vi "Get Target IP and Name.vi"(8 "error in (no error)":errorcluster, 11 "Item Ref in":T1 format="%.0x") -> (0 "error out":errorcluster, 1 "Name":string, 2 "IPAddress":string, 3 "Item Ref out":T1=18446744073709551615 format="%.0x")   [LabVIEW 2013, in "J1939 Addon System Explorer.lvlib"]
uses:
  <vilib>/NI Veristand/Custom Device API/Custom Device Item Ref.ctl
  NationalInstruments.VeriStand.SystemDefinitionAPI
  J1939 Addon System Explorer.lvlib
  <vilib>/NI Veristand/Custom Device Offline API/Custom Device Offline API.lvlib
  <vilib>/NI Veristand/Custom Device Tools/Custom Device Utility Library/Custom Device Utility Library.lvlib
  <vilib>/NI Veristand/Custom Device API/Custom Device API.lvlib
panel:
  # "OUTPUTS"
  # "INPUTS"
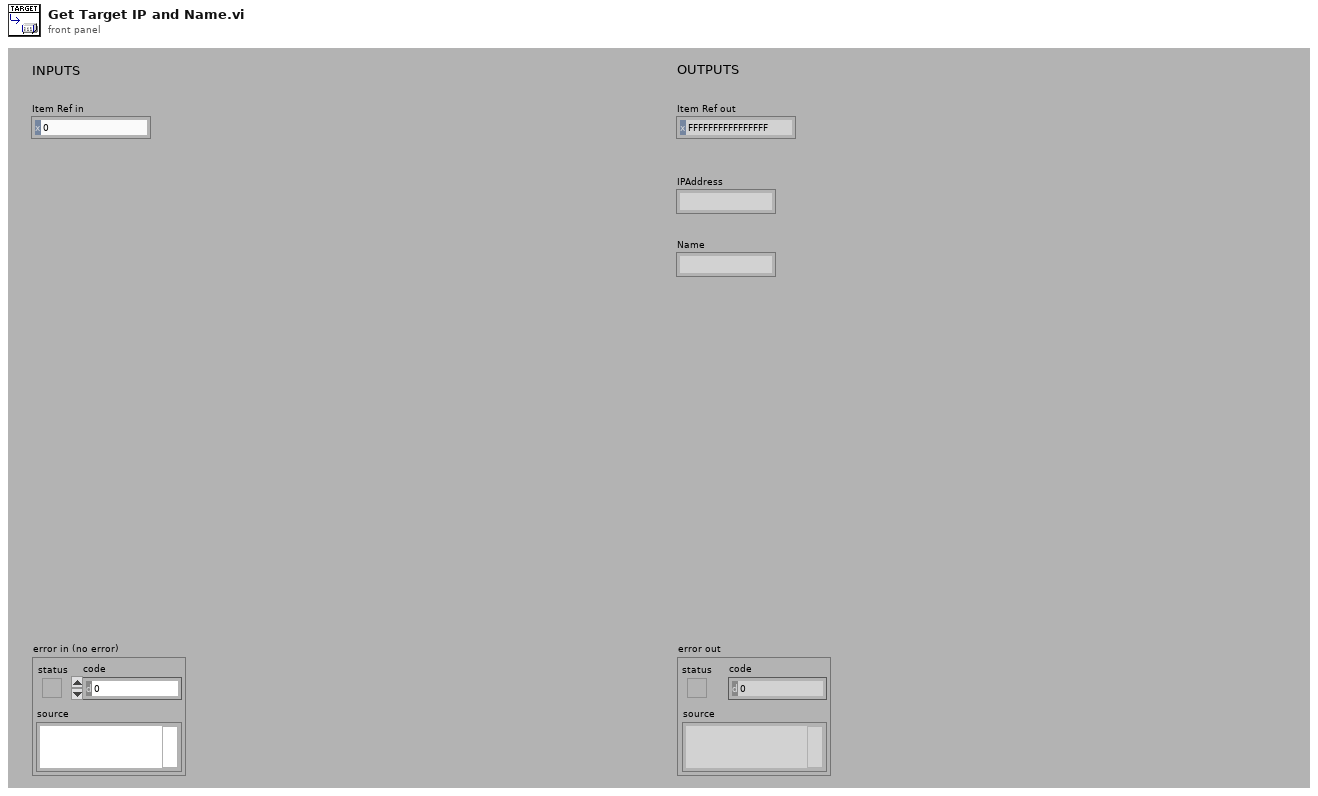
[diagram p1: front panel]
types:
  T1 = typedef "Custom Device API.lvlib/Custom Device Item Ref.ctl" = u64
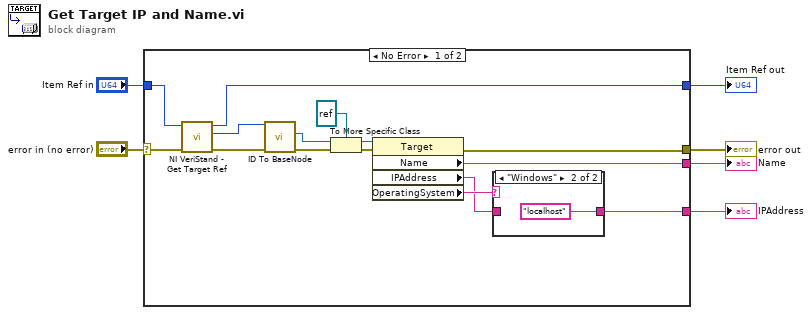
[diagram p0: block diagram]
diagram:
  n1 = case shown="No Error" "error in (no error)" {
    selector: "error in (no error)" -> [w18 w25]
    tunnel: [w12 w25] -> w5
    tunnel: "Item Ref in" -> [w19 w24]
    tunnel: [w11 _] -> w3
    tunnel: [w7 _] -> w2
    tunnel: [w10 w24] -> w1
    frame No Error {
      n2 = call <vilib>:"NI VeriStand - Get Target Ref.vi"("error in"=w18, "Item Ref in"=w19) -> ("error out"=w20:errorcluster, "Target Ref"=w21:T1, "Item Ref out"=w10:T1)  [unwired: 6 in, 1 out]
      n3 = call <vilib>:"ID To BaseNode.vi"("error in (no error)"=w20, "ID in"=w21) -> ("error out"=w13:errorcluster, "BaseNode"=w14:refnum<k24>)  [unwired: 7 in, 1 out]
      n4 = To More Specific Class(target class=refnum<k24> refnum, reference=w14, error in=w13) -> (specific class reference=w16:refnum<k24>, error out=w17:errorcluster)
      n5 = property class="Target"(reference=w16, error in=w17) -> (error out=w12:errorcluster, "Name"=w11:string, "IPAddress"=w8:string, "OperatingSystem"=w9:string)  [unwired: 1 out]
      n6 = case shown="\"Windows\"" w9 {
        tunnel: [w22 "localhost" ("IPAddress")] -> w7
        tunnel: w8 -> [w22 _]
        frame Default {
        }
        frame "Windows" {
        }
      }
    }
    frame Error {
    }
  }
  "error out" <- w5
  "Name" <- w3
  "IPAddress" <- w2
  "Item Ref out" <- w1
